vi "Get_Values.vi"(0 "reference in":refnum<class "Sig_Digital.lvclass">, 11 "error in (no error)":errorcluster) -> (4 "reference out":refnum<class "Sig_Digital.lvclass">, 6 "EU":bool, 8 "RAW":bool, 15 "error out":errorcluster)   [LabVIEW 2019, in "Sig_Digital.lvclass"]
uses:
  Sig_Digital.lvclass
  Sig_Digital.lvclass/Sig_Digital.ctl
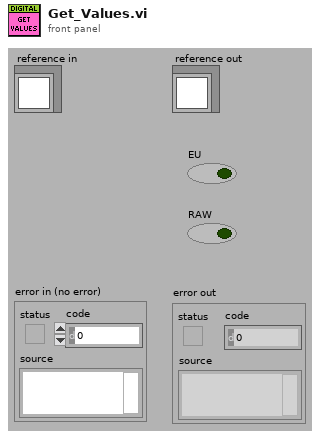
[diagram p1: front panel]
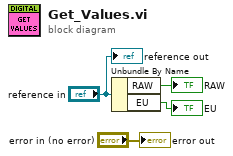
[diagram p0: block diagram]
diagram:
  n1 = Unbundle By Name("reference in") -> ("RAW"=→"RAW":bool, "EU"=→"EU":bool)
  "error out" <- "error in (no error)"
  "reference out" <- "reference in"
